vi "Write Voltage.vi"(8 "error in":errorcluster, 10 "Voltage":dbl, 11 "IF_XX in":refnum<class "IF_XX.lvclass">) -> (0 "error out":errorcluster, 3 "IF_XX out":refnum<class "IF_XX.lvclass">)   [LabVIEW 2019, in "IF_XX.lvlib" / "IF_XX.lvclass"]
doc: "Transmit the voltage setpoint command to the IF-XX\n\nThe example shows a readback operation, so I'm including the readback indicator for analysis during integration testing."
uses:
  Library/IF_XX.lvclass
  C:/Users/Public/Documents/Development/builds/Instruments/PowerSupply.lvlibp/Library/PowerSupply.lvclass
  Library/IF_XX.lvclass/IF_XX.ctl
  builds/Instruments/PowerSupply.lvlibp/Library/PowerSupply.lvclass
panel:
  out "Read data":string
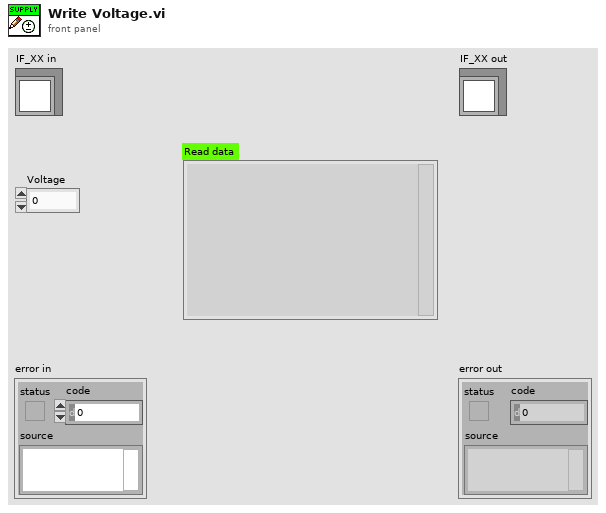
[diagram p1: front panel]
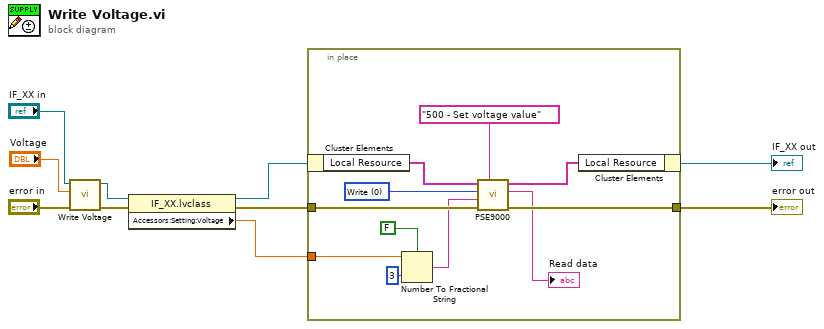
[diagram p0: block diagram]
diagram:
  n1 = call-parent "Write Voltage.vi"("error in"="error in", "Voltage"="Voltage", "PowerSupply in"="IF_XX in") -> ("error out"=w10:errorcluster, "PowerSupply out"=w6:refnum<class "IF_XX.lvclass">)  [unwired: 7 in]
  n2 = property class="IF_XX.lvclass"(reference=w6, error in=w10) -> (reference out=w5:refnum<class "IF_XX.lvclass">, error out=w3:errorcluster, "Accessors:Setting:Voltage"=w1:dbl)
  n3 = in-place {
    in-place-border: w3 -> [w21]
    in-place-border: [w20] -> w2
    in-place-border: w1 -> [w14]
    w12 = u8 0 items=["Write", "Read"] ("Access")
    n4 = in-place-cluster #1(w5) -> ("Local Resource"=w19:string[])
    n5 = Number To Fractional String(use system decimal point (T)=FALSE, number=w14, precision (6)=i16 3 ("Genauigkeit (6)")) -> (F-format string=w13:string)  [unwired: 1 in]
    n6 = call <instrlib>:"PSE9000.vi"("Command list"="500 - Set voltage value", "Error in"=w21, "Value"=w13, "Access"=w12, "Device information in"=w19) -> ("Error out"=w20:errorcluster, "Read data"=→"Read data":string, "Device information out"=w18:string[])  [unwired: 1 in, 1 out]
    n7 = in-place-cluster #1("Local Resource"=w18) -> (→"IF_XX out":refnum<class "IF_XX.lvclass">)
  }
  "error out" <- w2
